vi "EnviaDrive.vi"(6 "run":dbl, 7 "notificacao rapida in":string, 8 "tensao in":dbl[](array[numeric]), 9 "counts in":dbl[](array[numeric]), 10 "Chave de Acesso ao Drive":path, 11 "size":i32) -> (0 "Error":bool, 1 "notificacao rapida out":string)   [LabVIEW 2018]
uses:
  <vilib>/National Instruments/GDrive for LabVIEW/VIs/GDrive.lvlib
panel:
  in  "texto":string
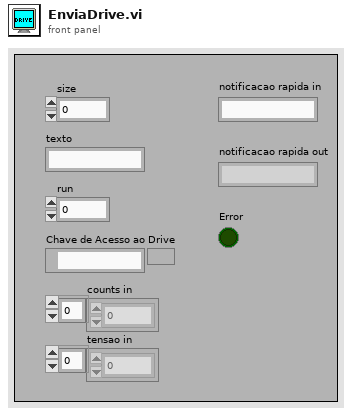
[diagram p1: front panel]
types:
  T1 = enum16{"open", "replace", "create", "open or create", "replace or create", "replace or create with confirmation"}
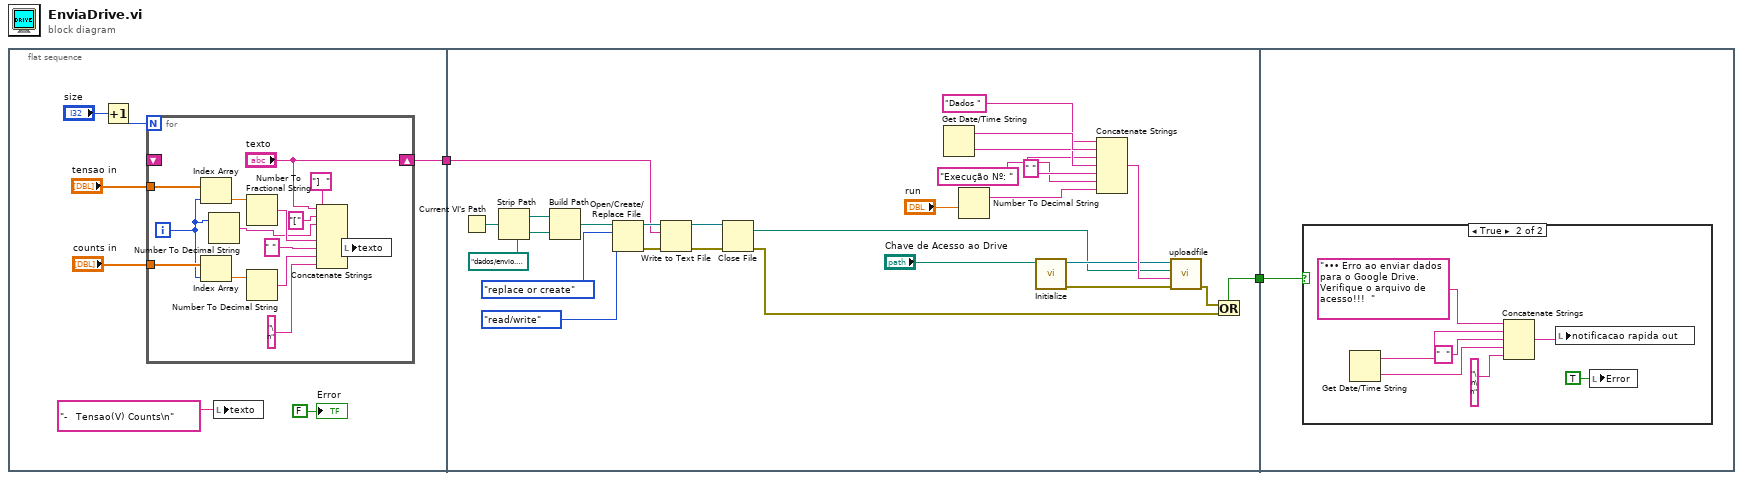
[diagram p0: block diagram]
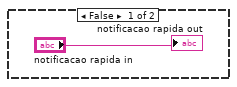
[diagram p2: hidden frame]
diagram:
  n1 = flat-sequence {
    tunnel: [w7] -> w2
    tunnel: w2 -> [w30]
    tunnel: [w24] -> w1
    tunnel: w1 -> [w50]
    frame #0 {
      n2 = Increment(x="size") -> (x+1=w8:i32)
      n3 = for {
        N: w8 -> [_]
        tunnel: "tensao in" -> [w23]
        tunnel: "counts in" -> [w20]
        shift-right: ["texto"] -> w7
        shift-left: _ -> [_]
        i -> [w12]
        n4 = Index Array(array=w23, index=w12) -> (element=w22:dbl)
        n5 = Index Array(array=w20, index=w12) -> (element=w16:dbl)
        n6 = Number To Decimal String(number=w12) -> (decimal integer string=w11:string)  [unwired: 1 in]
        n7 = Number To Fractional String(number=w22) -> (F-format string=w19:string)  [unwired: 3 in]
        n8 = Number To Decimal String(number=w16) -> (decimal integer string=w15:string)  [unwired: 1 in]
        n9 = Concatenate Strings("texto", "[" ("string"), w11, "]  " ("string"), w19, " " ("string"), w15, "\n" ("string")) -> (w21:string)
        n10 = local write "texto"(w21) -> ()
      }
      n11 = local write "texto"("-   Tensao(V) Counts\n" ("String")) -> ()
      "Error" <- FALSE ("Error")
    }
    frame #1 {
      w26 = " " ("string")
      n12 = Current VI's Path() -> (path=w34:path)
      n13 = Strip Path(path=w34) -> (stripped path=w35:path)  [unwired: 1 out]
      n14 = Build Path(base path=w35, name or relative path=path "dados/envio.txt" ("Path to Secret Client JSON")) -> (appended path=w33:path)
      n15 = Open/Create/Replace File(file path (use dialog)=w33, operation (0:open)=T1."replace or create", access (0:read/write)=enum16{"read/write", "read-only", "write-only"}."read/write") -> (refnum out=w42:refnum<file>, error out=w41:errorcluster)  [unwired: 3 in, 1 out]
      n16 = Write to Text File(file (use dialog)=w42, text=w30, error in=w41) -> (refnum out=w38:refnum<file>, error out=w39:errorcluster)  [unwired: 1 in, 1 out]
      n17 = Close File(refnum=w38, error in=w39) -> (path=w40:path, error out=w48:errorcluster)
      n18 = Get Date/Time String() -> (date string=w37:string, time string=w36:string)  [unwired: 3 in]
      n19 = Number To Decimal String(number="run") -> (decimal integer string=w46:string)  [unwired: 1 in]
      n20 = call <vilib>:"Initialize.vi"("Path to Secret Client JSON"="Chave de Acesso ao Drive") -> ("error out"=w43:errorcluster, "Google Drive Service Ref"=w44:refnum<k24>)  [unwired: 9 in]
      n21 = Concatenate Strings("Dados " ("File Name on Drive"), w37, w26, w36, w26, "Execução Nº: " ("string"), w46) -> (w45:string)
      n22 = call <vilib>:"uploadfile.vi"("error in (no error)"=w43, "File Name on Drive"=w45, "Local Path"=w40, "Google Drive Service Ref"=w44) -> ("error out"=w49:errorcluster)  [unwired: 6 in]
      n23 = Or(x=w49, y=w48) -> (x .or. y?=w24:bool)
    }
    frame #2 {
      n24 = case shown="True" w50 {
        frame False {
          "notificacao rapida out" <- "notificacao rapida in"
        }
        frame True {
          n25 = Get Date/Time String() -> (date string=w56:string, time string=w53:string)  [unwired: 3 in]
          n26 = Concatenate Strings("••• Erro ao enviar dados para o Google Drive. Verifique o arquivo de acesso!!!  " ("String 3"), w56, "  " ("string"), w53, "\n\n" ("string")) -> (w55:string)
          n27 = local write "notificacao rapida out"(w55) -> ()
          n28 = local write "Error"(TRUE ("Error")) -> ()
        }
      }
    }
  }
